vi "Read FPGA FIFO MTi.vi"(6 "Error In":errorcluster, 9 "Vessel.lvclass":refnum<class "Vessel.lvclass">) -> (0 "Error Out":errorcluster, 3 "Vessel.lvclass 2":refnum<class "Vessel.lvclass">)   [LabVIEW 2014, in "Vessel.lvclass"]
uses:
  Vessel.lvclass
  <vilib>/rvi/interface/nirviMethod/nirviMethod.xnode
  cRIO/FPGA/9870 Interface DMA (FPGA).vi
  <vilib>/rvi/errors/niLvFpgaMergeErrorWithErrorCode.vi
  FPGA Bitfiles/MinervaControlSy_FPGATarget_9870InterfaceDMA_4D1233B8.lvbitx
  <vilib>/FPGAPlugInAG/cRIO-9074/niLvFpga_ReadFifo_cRIO-9074.vi
panel:
  out "MT_DATA":sgl[](array[numeric])
  out "MT_BITS":u8[](array[numeric])
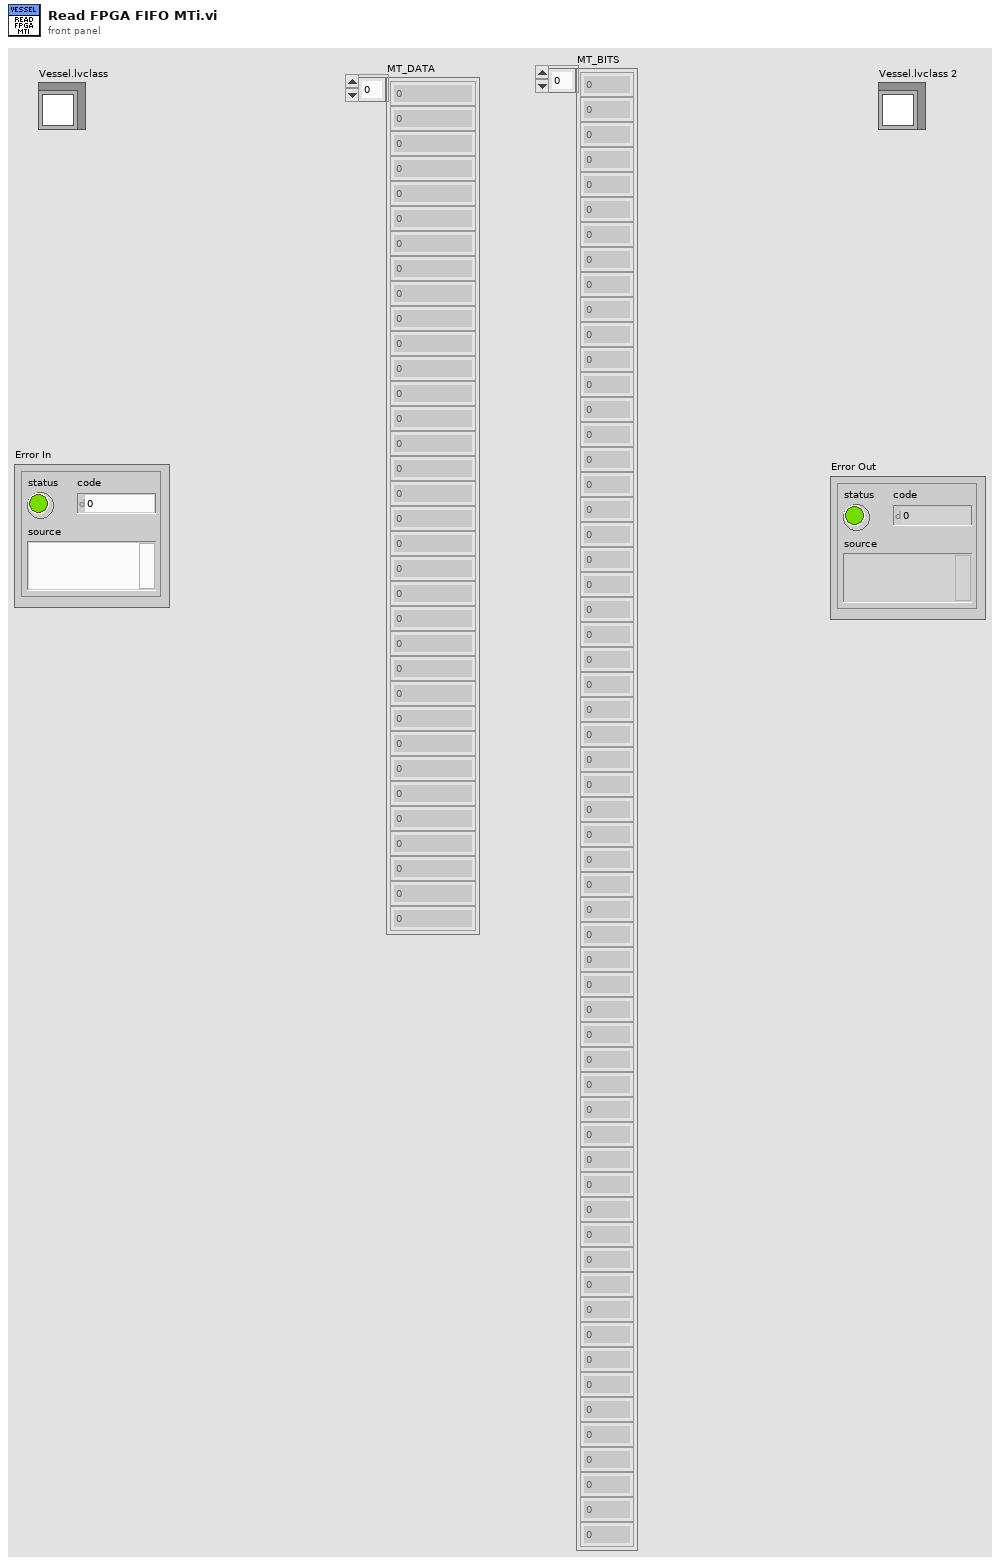
[diagram p1: front panel]
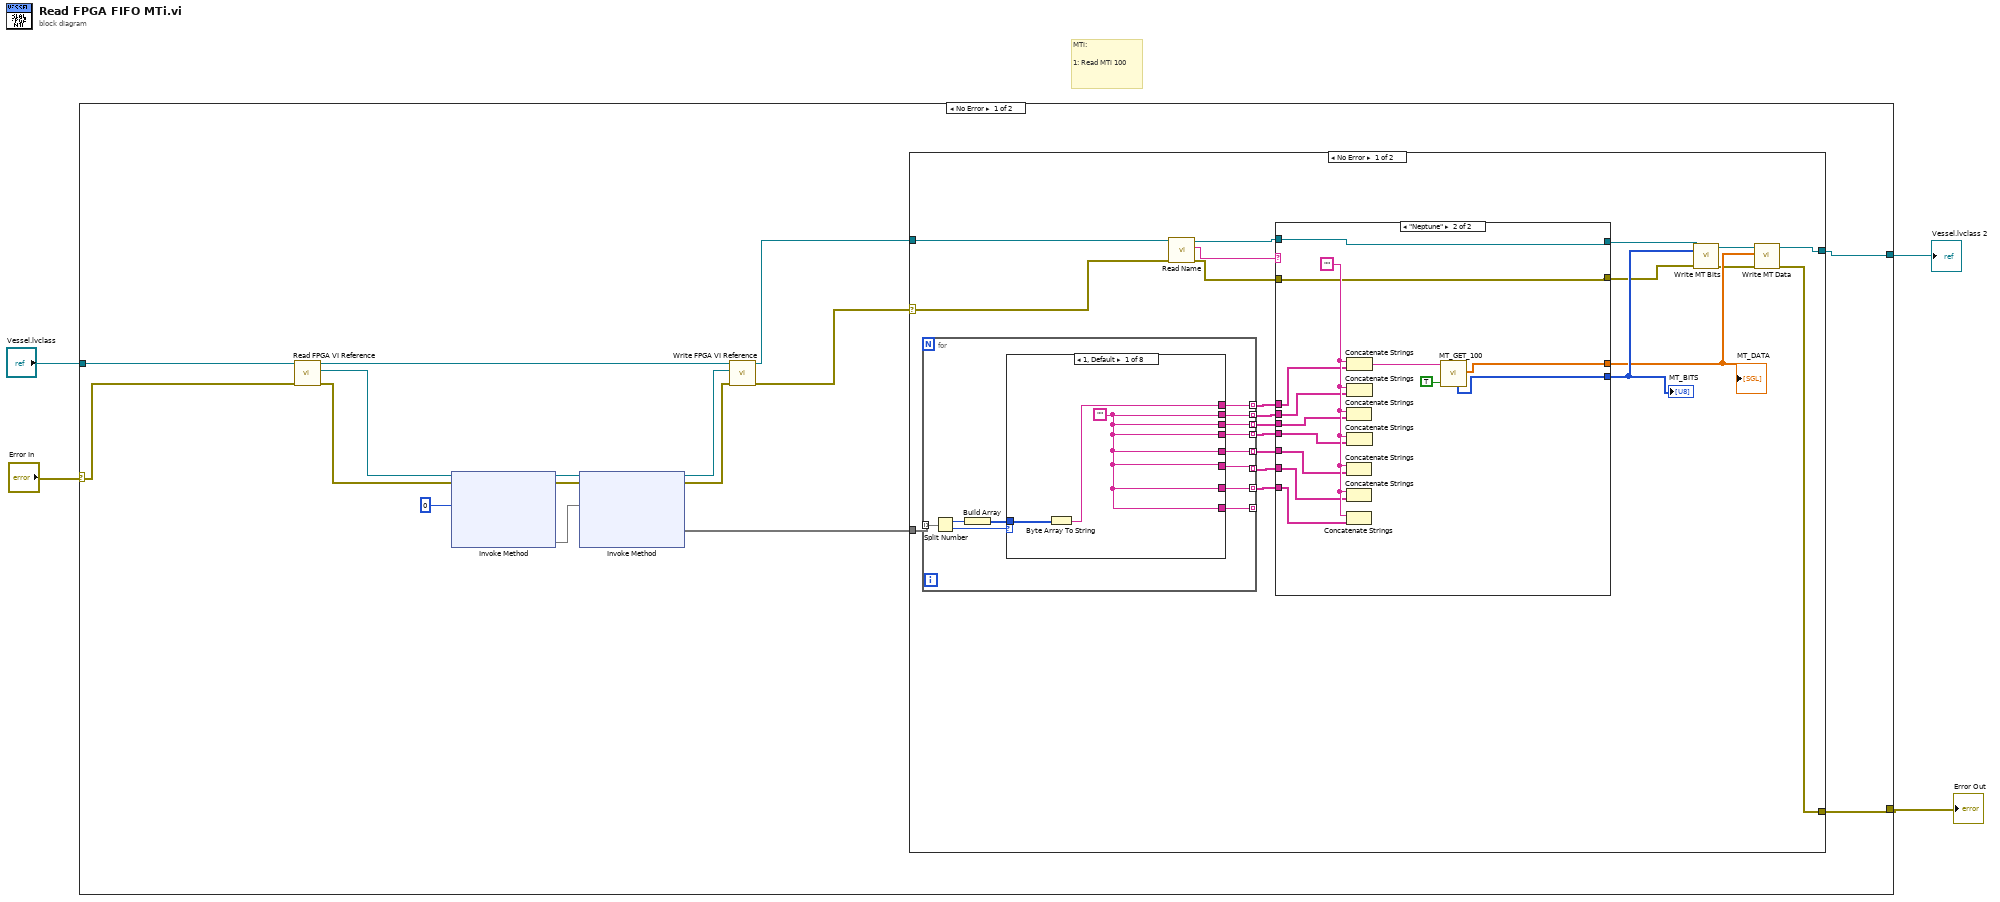
[diagram p0: block diagram]
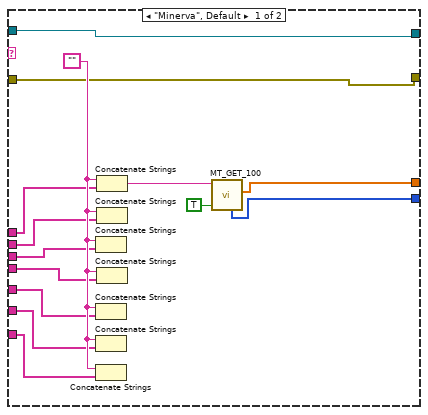
[diagram p2: hidden frame]
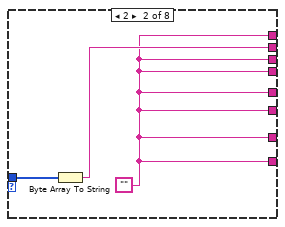
[diagram p3: hidden frame]
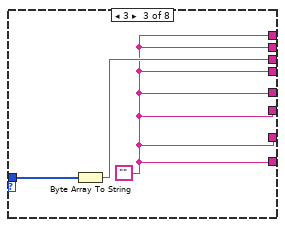
[diagram p4: hidden frame]
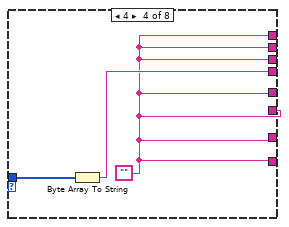
[diagram p5: hidden frame]
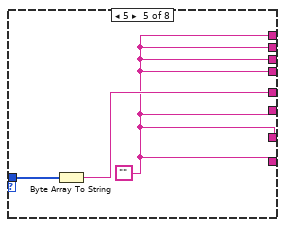
[diagram p6: hidden frame]
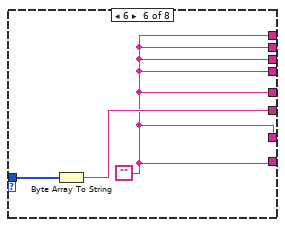
[diagram p7: hidden frame]
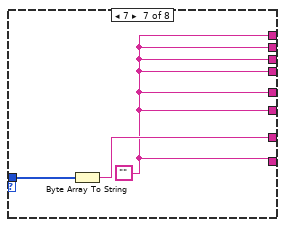
[diagram p8: hidden frame]
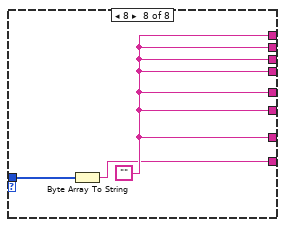
[diagram p9: hidden frame]
diagram:
  # "MTi:\n\n1: Read MTi 100"
  n1 = case shown="No Error" "Error In" {
    selector: "Error In" -> [w7 w108]
    tunnel: "Vessel.lvclass" -> [w8 w109]
    tunnel: [w13 w108] -> w2
    tunnel: [w12 w109] -> w1
    frame No Error {
      n2 = call-dynamic "Read FPGA VI Reference.vi"("error in (no error)"=w7, "Vessel in"=w8) -> ("error out"=w5:errorcluster, "FPGA VI Reference Out"=w9:refnum<k20>, "Vessel out"=w6:refnum<class "Vessel.lvclass">)  [unwired: 7 in]
      n3 = xnode "Invoke Method"("FPGA VI Reference In"=w9, "error in"=w5, "Number of Elements"=u32 0) -> ("FPGA VI Reference Out"=w17:refnum<k20>, "error out"=w18:errorcluster, "Elements Remaining"=w20)  [unwired: 1 in, 1 out]
      n4 = xnode "Invoke Method"("FPGA VI Reference In"=w17, "error in"=w18, "Number of Elements"=w20) -> ("FPGA VI Reference Out"=w15:refnum<k20>, "error out"=w14:errorcluster, "Data"=w16:void[])  [unwired: 1 in, 1 out]
      n5 = call-dynamic "Write FPGA VI Reference.vi"("error in (no error)"=w14, "FPGA VI Reference Out 2"=w15, "Vessel in"=w6) -> ("error out"=w10:errorcluster, "Vessel out"=w11:refnum<class "Vessel.lvclass">)  [unwired: 7 in]
      n6 = case shown="No Error" w10 {
        selector: w10 -> [w23 w107]
        tunnel: w16 -> [w38 _]
        tunnel: [w24 w107] -> w13
        tunnel: w11 -> [w31 w106]
        tunnel: [w27 w106] -> w12
        frame No Error {
          n7 = for {
            tunnel: w38 -> [w75] mode=indexing
            tunnel: [w79] -> w39 mode=indexing
            tunnel: [w78] -> w40 mode=indexing
            tunnel: [w77] -> w36 mode=indexing
            tunnel: [w76] -> w41 mode=indexing
            tunnel: [w73] -> w37 mode=indexing
            tunnel: [w72] -> w35 mode=indexing
            tunnel: [w71] -> w34 mode=indexing
            tunnel: [w70] -> _ mode=indexing
            n8 = Split Number(x=w75) -> (hi(x)=w81:u16, lo(x)=w80:u16)
            n9 = Build Array(w81) -> (w74:u16[])
            n10 = case shown="1, Default" w80 {
              tunnel: [w83 w85 w88 w91 w94 w97 w100 w104] -> w79
              tunnel: [w82 w86 w88 w91 w94 w97 w100 w104] -> w78
              tunnel: [w82 w85 w89 w91 w94 w97 w100 w104] -> w77
              tunnel: [w82 w85 w88 w92 w94 w97 w100 w104] -> w76
              tunnel: w74 -> [w84 w87 w90 w93 w96 w99 w102 w105]
              tunnel: [w82 w85 w88 w91 w95 w97 w100 w104] -> w73
              tunnel: [w82 w85 w88 w91 w94 w98 w100 w104] -> w72
              tunnel: [w82 w85 w88 w91 w94 w97 w101 w104] -> w71
              tunnel: [w82 w85 w88 w91 w94 w97 w100 w103] -> w70
              frame 1, Default {
                w82 = ""
                n11 = Byte Array To String(unsigned byte array=w84) -> (string=w83:string)
              }
              frame 2 {
                w85 = ""
                n12 = Byte Array To String(unsigned byte array=w87) -> (string=w86:string)
              }
              frame 3 {
                w88 = ""
                n13 = Byte Array To String(unsigned byte array=w90) -> (string=w89:string)
              }
              frame 4 {
                w91 = ""
                n14 = Byte Array To String(unsigned byte array=w93) -> (string=w92:string)
              }
              frame 5 {
                w94 = ""
                n15 = Byte Array To String(unsigned byte array=w96) -> (string=w95:string)
              }
              frame 6 {
                w97 = ""
                n16 = Byte Array To String(unsigned byte array=w99) -> (string=w98:string)
              }
              frame 7 {
                w100 = ""
                n17 = Byte Array To String(unsigned byte array=w102) -> (string=w101:string)
              }
              frame 8 {
                w104 = ""
                n18 = Byte Array To String(unsigned byte array=w105) -> (string=w103:string)
              }
            }
          }
          n19 = call-dynamic "Read Name.vi"("error in (no error)"=w23, "Vessel in"=w31) -> ("error out"=w22:errorcluster, "Name"=w32:string, "Vessel out"=w33:refnum<class "Vessel.lvclass">)  [unwired: 7 in]
          n20 = case shown="\"Neptune\"" w32 {
            tunnel: w41 -> [w51 w65]
            tunnel: w40 -> [w53 w67]
            tunnel: w39 -> [w54 w68]
            tunnel: w37 -> [w50 w64]
            tunnel: w36 -> [w52 w66]
            tunnel: w35 -> [w49 w63]
            tunnel: w33 -> [w46 w60]
            tunnel: w34 -> [w48 w62]
            tunnel: [w46 w60] -> w30
            tunnel: [w45 w59] -> w29
            tunnel: [w44 w58] -> w26
            tunnel: w22 -> [w42 w56]
            tunnel: [w42 w56] -> w21
            frame "Minerva", Default {
              w55 = ""
              n21 = Concatenate Strings(w55, w52) -> ()  [unwired: 1 out]
              n22 = Concatenate Strings(w55, w50) -> ()  [unwired: 1 out]
              n23 = Concatenate Strings(w55, w49) -> ()  [unwired: 1 out]
              n24 = Concatenate Strings(w55, w48) -> ()  [unwired: 1 out]
              n25 = Concatenate Strings(w55, w54) -> (w43:string)
              n26 = Concatenate Strings(w55, w53) -> ()  [unwired: 1 out]
              n27 = Concatenate Strings(w55, w51) -> ()  [unwired: 1 out]
              n28 = call "MT_GET_100.vi"("Use checksum"=TRUE, "read buffer"=w43) -> ("MT_DATA"=w44:sgl[], "MT_BITS"=w45:u8[])  [unwired: 6 in, 2 out]
            }
            frame "Neptune" {
              w69 = ""
              n29 = Concatenate Strings(w69, w66) -> ()  [unwired: 1 out]
              n30 = Concatenate Strings(w69, w64) -> ()  [unwired: 1 out]
              n31 = Concatenate Strings(w69, w63) -> ()  [unwired: 1 out]
              n32 = Concatenate Strings(w69, w62) -> ()  [unwired: 1 out]
              n33 = Concatenate Strings(w69, w68) -> (w57:string)
              n34 = Concatenate Strings(w69, w67) -> ()  [unwired: 1 out]
              n35 = Concatenate Strings(w69, w65) -> ()  [unwired: 1 out]
              n36 = call "MT_GET_100.vi"("Use checksum"=TRUE, "read buffer"=w57) -> ("MT_DATA"=w58:sgl[], "MT_BITS"=w59:u8[])  [unwired: 6 in, 2 out]
            }
          }
          "MT_BITS" <- w29
          "MT_DATA" <- w26
          n37 = call-dynamic "Write MT Bits.vi"("error in (no error)"=w21, "MT Bits"=w29, "Vessel in"=w30) -> ("error out"=w25:errorcluster, "Vessel out"=w28:refnum<class "Vessel.lvclass">)  [unwired: 7 in]
          n38 = call-dynamic "Write MT Data.vi"("error in (no error)"=w25, "MT Data"=w26, "Vessel in"=w28) -> ("error out"=w24:errorcluster, "Vessel out"=w27:refnum<class "Vessel.lvclass">)  [unwired: 7 in]
        }
        frame Error {
        }
      }
    }
    frame Error {
    }
  }
  "Vessel.lvclass 2" <- w1
  "Error Out" <- w2
